vi "GoalieChute.vi"(6 "Current State":dbl=1.0, 8 "balls":T5[](array[typedef])=[{"x"=-974.5169677734375, "y"=-3444.3310546875, "timestamp"=timestamp(2082759045.994995 s since 1904-01-01), "Vel_x"=0.0, "Vel_y"=0.0}], 9 "Field Size in":T6={"line_width"=10, "field_length"=9000, "field_width"=6000, "boundary_width"=250, "referee_width"=425, "goal_width"=700, "goal_depth"=180, "goal_wall_width"=20, "center_circle_radius"=500, "defense_radius"=500, "defense_stretch"=350, "free_kick_from_defense_dist"=700, "penalty_spot_from_field_line_dist"=450, "penalty_line_from_spot_dist"=350}, 10 "Robot in":T2={"id"=5, "function"=enum."Attacker", "x"=-983.1382446289062, "y"=-3000.010498046875, "orientation"=-1.5516623258590698, "v_tangent"=0.0, "v_normal"=0.0, "v_ang"=0.0, "kick_x"=0.0, "kick_z"=0.0, "dribble"=FALSE, "Timestamp"=timestamp(2082759045.994995 s since 1904-01-01), "dest_x"=0.0, "dest_y"=0.0, "dest_orientation"=0.0, "estimatives"={"est_v_tangent"=0.0, "est_v_normal"=0.0, "est_vx"=0.0, "est_vy"=0.0}, "dest_x_kick"=0.0, "dest_y_kick"=0.0, "Gap Coord"=[], "States"=enum."GoToTangent"}, 11 "IA State Input 2":T1={"our_robots"=[], "enemy_robots"=[], "balls"=[], "geometry"={"line_width"=0, "field_length"=0, "field_width"=0, "boundary_width"=0, "referee_width"=0, "goal_width"=0, "goal_depth"=0, "goal_wall_width"=0, "center_circle_radius"=0, "defense_radius"=0, "defense_stretch"=0, "free_kick_from_defense_dist"=0, "penalty_spot_from_field_line_dist"=0, "penalty_line_from_spot_dist"=0}, "IA Judge"={"stage"="", "command"="", "our_goalie_id"=0.0, "enemy_goalie_id"=0.0, "command\nenum"=enum."Halt", "Time"=enum."Azul"}, "Received Timestamp"=timestamp(0 s since 1904-01-01), "Events"={"Touch"=FALSE, "Ball out"=FALSE, "id touch"=0.0, "Ball out of \nVision"=FALSE, "Ball inside \nGoalie area"=FALSE, "Robot not responding"=FALSE, "Robots responding status"=[1.0, 1.0, 1.0, 1.0, 1.0, 1.0], "Enemy Ball \nPossession"=FALSE}}) -> (1 "Next State":dbl=1.0, 2 "Robot out":T2={"id"=5, "function"=enum."Attacker", "x"=-983.1382446289062, "y"=-3000.010498046875, "orientation"=-1.5516623258590698, "v_tangent"=0.0001540345015520423, "v_normal"=0.008599927144915481, "v_ang"=0.002668461263266586, "kick_x"=0.0, "kick_z"=0.0, "dribble"=FALSE, "Timestamp"=timestamp(2082759045.994995 s since 1904-01-01), "dest_x"=0.0, "dest_y"=0.0, "dest_orientation"=0.0, "estimatives"={"est_v_tangent"=0.0, "est_v_normal"=0.0, "est_vx"=0.0, "est_vy"=0.0}, "dest_x_kick"=0.0, "dest_y_kick"=0.0, "Gap Coord"=[], "States"=enum."GoToTangent"})   [LabVIEW 2016]
uses:
  Core/AI Robot.ctl
  Functions Enum.ctl
  AttackerStates.ctl
  Core/Field Size.ctl
  Core/AI Ball.ctl
  Core/AI Input.ctl
  Core/AI Judge.ctl
  Command Enum.ctl
  <vilib>/Analysis/coordinate.llb/2D Cartesian Coordinate Rotation (Scalar).vi
  <vilib>/Analysis/NI_AALPro.lvlib
panel:
  out "V_tangent":dbl(graph)
  out "Waveform Chart":dbl(graph)
  out "Elapsed Time (s)":dbl
  in  "Time Target \nto transition":dbl=1.0 caption="Time Target (s)"
  in  "Longe":dbl=300.0 format="%#_13g"
  out "bola fora?":bool=TRUE
  in  "Cone de chute":dbl=0.09 format="%#_13g"
  in  "Perto":dbl=300.0 format="%#_13g"
  in  "Cone de rotação":dbl=1.3 format="%#_13g"
  in  "min dist to kick":dbl=150.0 format="%#_13g"
  in  "Dist a frente da bola":dbl format="%#_13g"
  in  "raio da circunferencia":dbl=175.0 format="%#_13g"
  in  "distance between ball and robot":dbl=125.0 format="%#_13g"
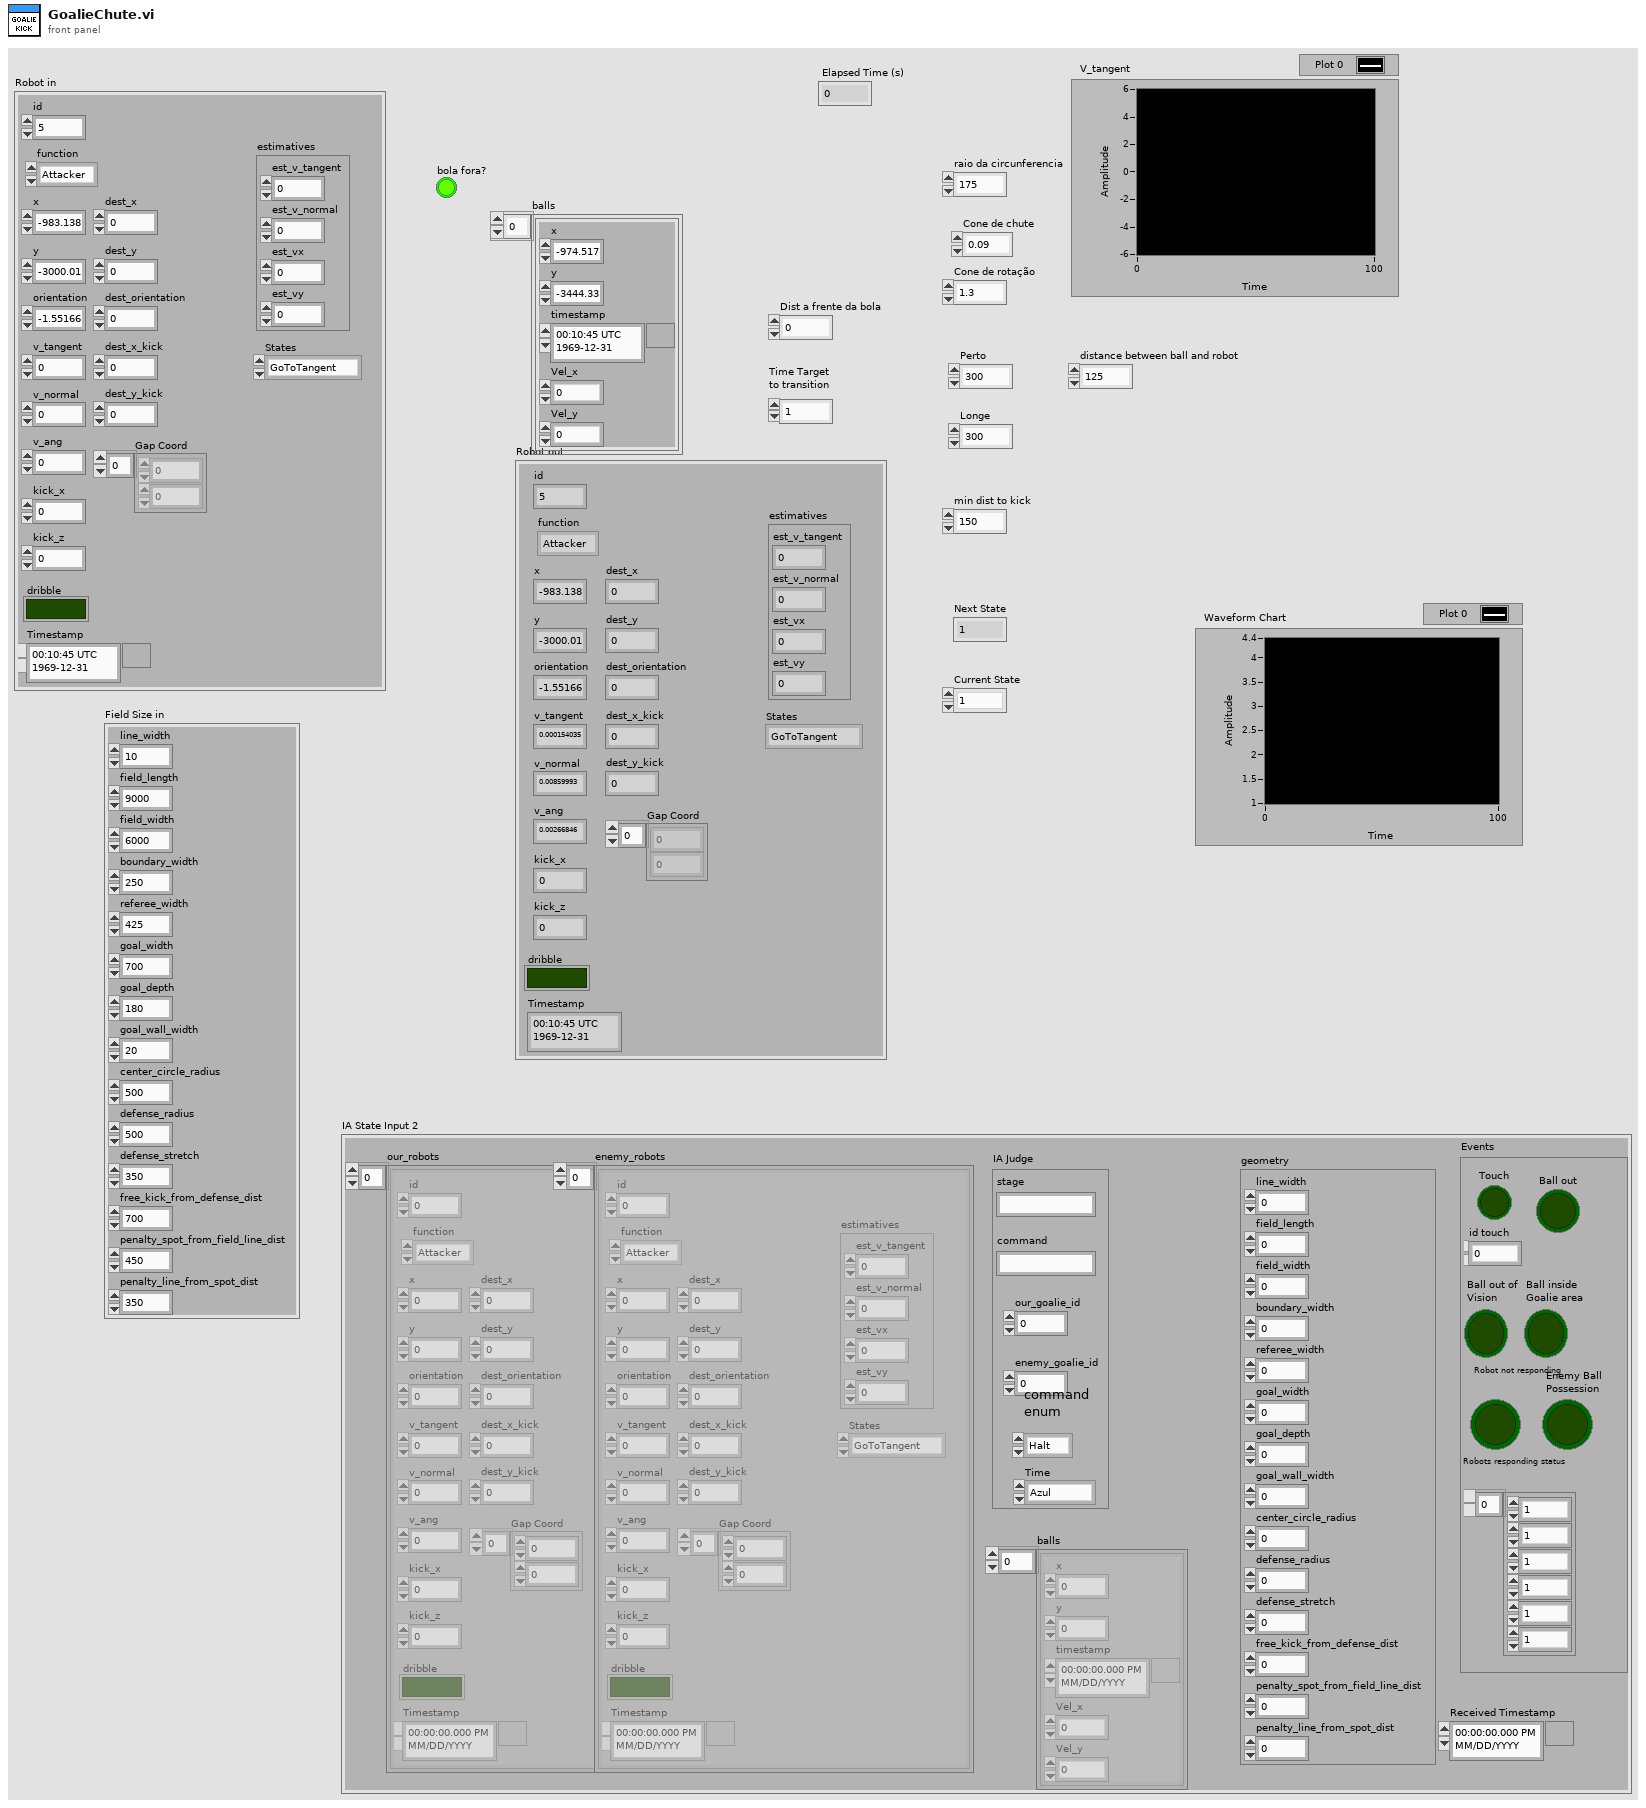
[diagram p1: front panel]
types:
  T1 = typedef "AI Input.ctl" = cluster{"our_robots":T2[], "enemy_robots":T2[], "balls":T5[], "geometry":T6, "IA Judge":T7, "Received Timestamp":timestamp, "Events":cluster{"Touch":bool, "Ball out":bool, "id touch":dbl, "Ball out of \nVision":bool, "Ball inside \nGoalie area":bool, "Robot not responding":bool, "Robots responding status":dbl[], "Enemy Ball \nPossession":bool}}
  T2 = typedef "AI Robot.ctl" = cluster{"id":u32, "function":T3, "x":dbl, "y":dbl, "orientation":dbl, "v_tangent":dbl, "v_normal":dbl, "v_ang":dbl, "kick_x":dbl, "kick_z":dbl, "dribble":bool, "Timestamp":timestamp, "dest_x":dbl, "dest_y":dbl, "dest_orientation":dbl, "estimatives":cluster{"est_v_tangent":dbl, "est_v_normal":dbl, "est_vx":dbl, "est_vy":dbl}, "dest_x_kick":dbl, "dest_y_kick":dbl, "Gap Coord":dbl[], "States":T4}
  T3 = typedef "Functions Enum.ctl" = enum16{"Attacker", "Goalie", "Defender", "Striker", "Goto 0", "Dummy", "Kicker", "ZigZag"}
  T4 = typedef "AttackerStates.ctl" = enum16{"Pass", "GoToTangent", "BallGetting", "GoToKick", ""}
  T5 = typedef "AI Ball.ctl" = cluster{"x":dbl, "y":dbl, "timestamp":timestamp, "Vel_x":dbl, "Vel_y":dbl}
  T6 = typedef "Field Size.ctl" = cluster{"line_width":u32, "field_length":u32, "field_width":u32, "boundary_width":u32, "referee_width":u32, "goal_width":u32, "goal_depth":u32, "goal_wall_width":u32, "center_circle_radius":u32, "defense_radius":u32, "defense_stretch":u32, "free_kick_from_defense_dist":u32, "penalty_spot_from_field_line_dist":u32, "penalty_line_from_spot_dist":u32}
  T7 = typedef "AI Judge.ctl" = cluster{"stage":string, "command":string, "our_goalie_id":dbl, "enemy_goalie_id":dbl, "command\nenum":T8, "Time":enum16{"Azul", "Amarelo"}}
  T8 = typedef "Command Enum.ctl" = enum16{"Halt", "Stop", "Force Start", "PKA Normal Start", "Prepare Kickoff Ally", "PKE Normal Start", "Prepare Kickoff Enemy", "Prepare Penalty Ally", "PPA Normal Start", "Prepare Penalty Enemy", "PPE Normal Start", "Direct Free Enemy", "Direct Free Ally", "Indirect Free Enemy", "Indirect Free Ally", "Timeout Enemy", "Timeout Ally", "Goal Enemy", "Goal Ally", "Ball Placement Enemy", "Ball Placement Ally", "Normal Half Time", "Extra Time Break", "Extra Half Time", "None"}
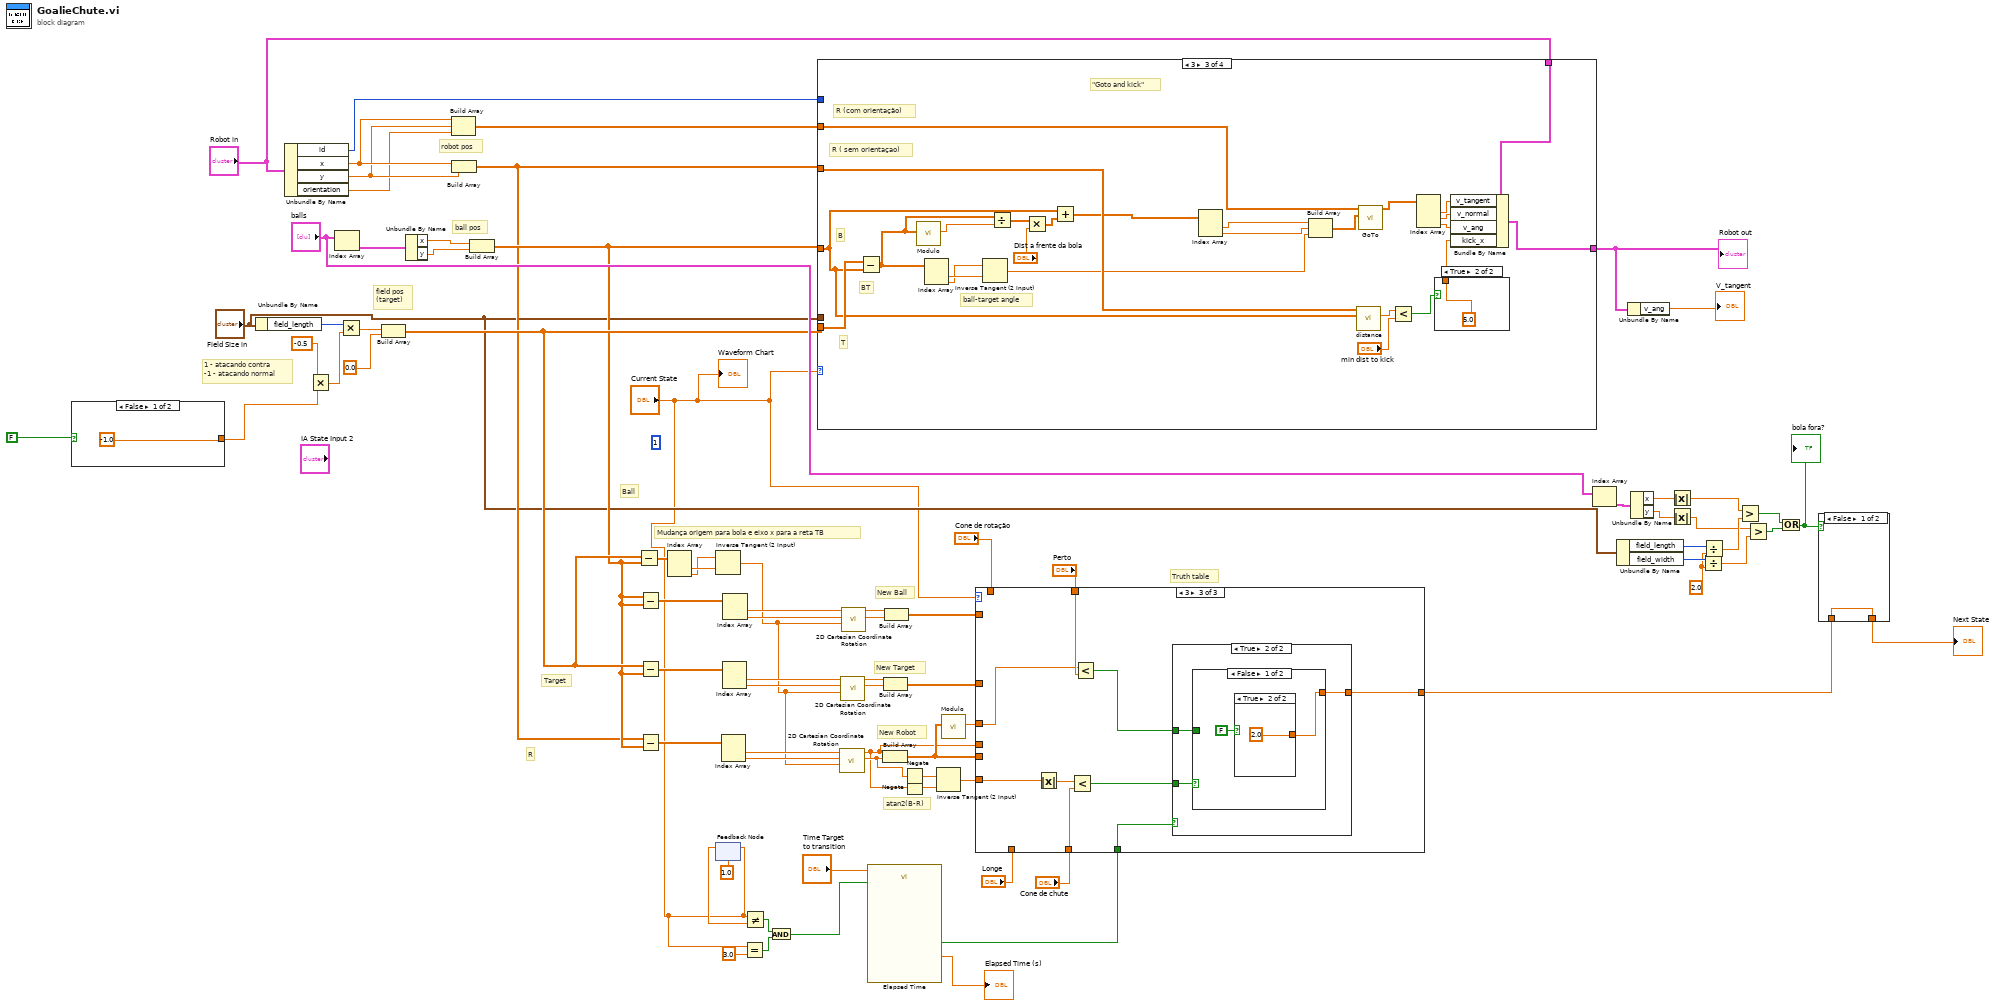
[diagram p0: block diagram]
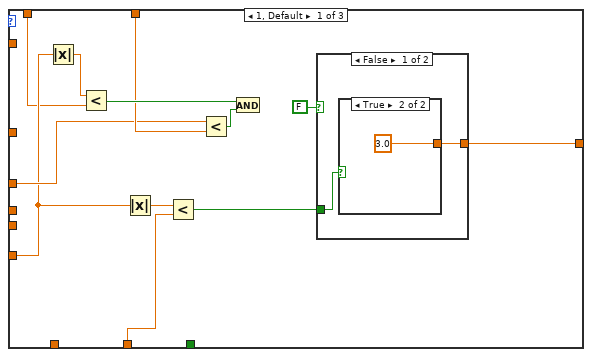
[diagram p2: hidden frame]
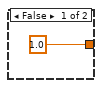
[diagram p3: hidden frame]
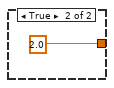
[diagram p4: hidden frame]
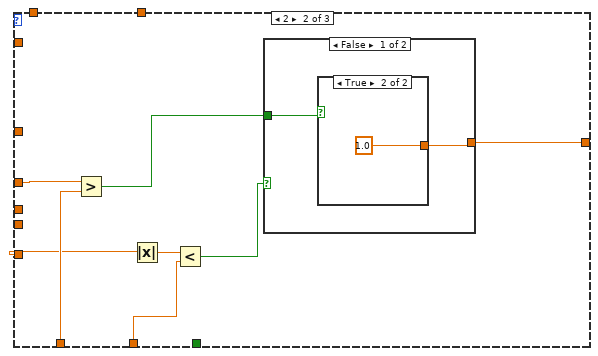
[diagram p5: hidden frame]
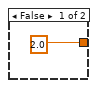
[diagram p6: hidden frame]
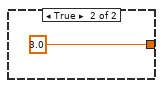
[diagram p7: hidden frame]
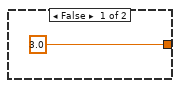
[diagram p8: hidden frame]
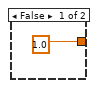
[diagram p9: hidden frame]
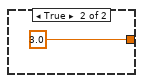
[diagram p10: hidden frame]
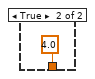
[diagram p11: hidden frame]
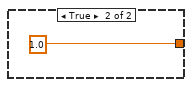
[diagram p12: hidden frame]
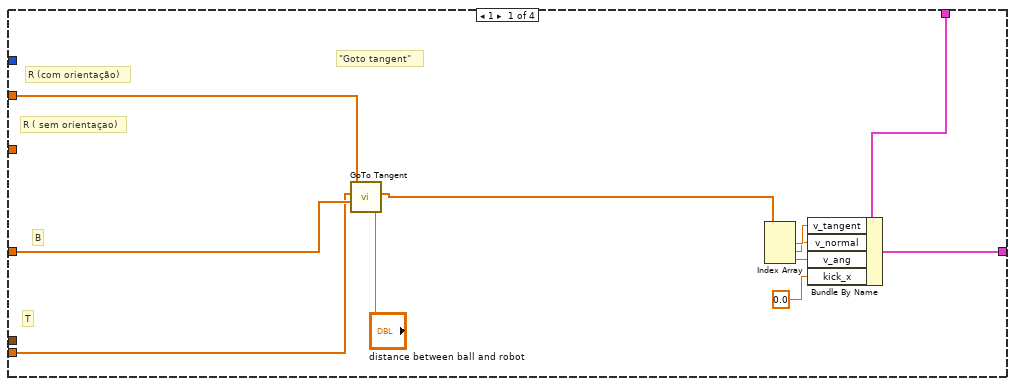
[diagram p13: hidden frame]
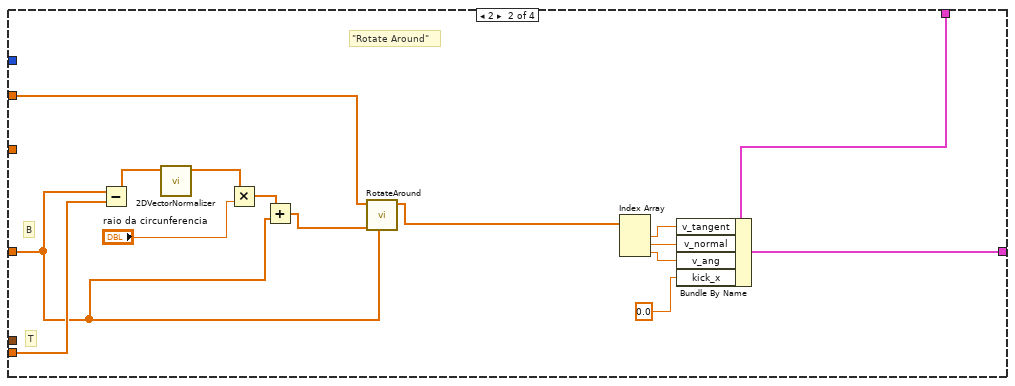
[diagram p14: hidden frame]
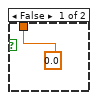
[diagram p15: hidden frame]
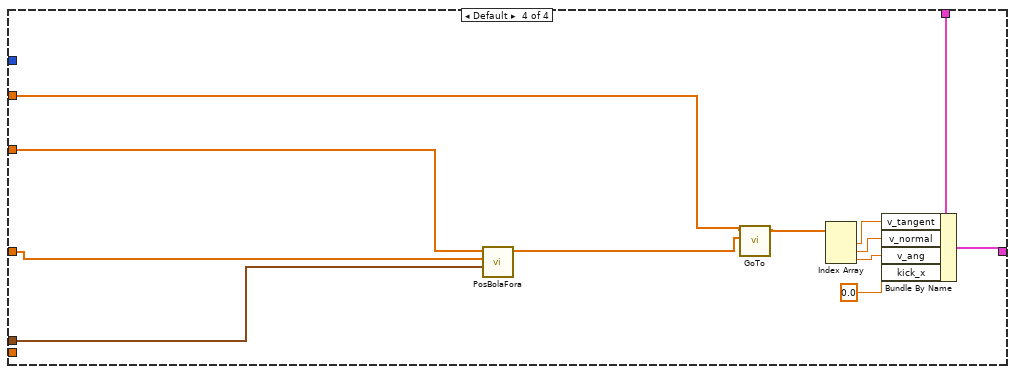
[diagram p16: hidden frame]
diagram:
  (unwired) 1
  w60 = 2.0 ("y")
  # "atan2(B-R)"
  # "New Robot"
  # "New Target"
  # "New Ball"
  # "R"
  # "Ball"
  # "Target"
  # "Mudança origem para bola e eixo x para a reta TB"
  # "1 - atacando contra\n-1 - atacando normal"
  # "Truth table"
  # "robot pos"
  # "field pos\n(target)"
  # "ball pos"
  n1 = case shown="False" FALSE {
    tunnel: [-1.0 ("attck contra? 2") 1.0] -> w22
    frame False {
    }
    frame True {
    }
  }
  n2 = Unbundle By Name("Field Size in") -> ("field_length"=w77:u32)
  n3 = Unbundle By Name("Robot in") -> ("id"=w16:u32, "x"=w73:dbl, "y"=w72:dbl, "orientation"=w69:dbl)
  n4 = Multiply(x=-0.5, y=w22) -> (x*y=w67:dbl)
  n5 = Index Array(array="balls") -> (element=w78:T5)  [unwired: 1 in]
  n6 = Multiply(x=w77, y=w67) -> (x*y=w76:dbl)
  n7 = Build Array(w76, 0.0 ("element")) -> (w34:dbl[])
  n8 = Unbundle By Name(w78) -> ("x"=w75:dbl, "y"=w74:dbl)
  n9 = Build Array(w73, w72, w69) -> (w70:dbl[])
  n10 = Build Array(w73, w72) -> (w32:dbl[])
  n11 = Build Array(w75, w74) -> (w33:dbl[])
  n12 = Subtract(x=w34, y=w33) -> (x-y=w42:dbl[])
  n13 = Subtract(x=w33, y=w33) -> (x-y=w49:dbl[])
  n14 = Subtract(x=w34, y=w33) -> (x-y=w46:dbl[])
  n15 = Subtract(x=w32, y=w33) -> (x-y=w43:dbl[])
  n16 = Index Array(array=w42) -> (element #1=w41:dbl, element #2=w40:dbl)  [unwired: 2 in]
  n17 = Inverse Tangent (2 Input)(1:w41, 2:w40) -> (0:w35:dbl)
  n18 = feedback #1(1.0 ("Current State")) -> (w8:dbl)
  n19 = feedback-in #1("Current State") -> ()
  n20 = Index Array(array=w43) -> (element #1=w45:dbl, element #2=w44:dbl)  [unwired: 2 in]
  n21 = Index Array(array=w46) -> (element #1=w48:dbl, element #2=w47:dbl)  [unwired: 2 in]
  n22 = Index Array(array=w49) -> (element #1=w51:dbl, element #2=w50:dbl)  [unwired: 2 in]
  n23 = Equal?(x="Current State", y=3.0) -> (x = y?=w12:bool)
  n24 = Not Equal?(x="Current State", y=w8) -> (x != y?=w11:bool)
  n25 = And(x=w11, y=w12) -> (x .and. y?=w6:bool)
  n26 = case shown="3" "Current State" {
    tunnel: [w91 w106 w132 w146] -> w4
    tunnel: "Robot in" -> [w90 w93 w131 w145]
    tunnel: w70 -> [w88 w105 w117 w137]
    tunnel: w32 -> [_ _ w126 w139]
    tunnel: w33 -> [w84 w92 w107 w140]
    tunnel: w34 -> [w83 w99 w123 _]
    tunnel: "Field Size in" -> [_ _ _ w138]
    tunnel: w16 -> [_ _ _ _]
    frame 1 {
      # "\"Goto tangent\""
      # "B"
      # "T"
      # "R ( sem orientaçao)"
      # "R (com orientação)"
      n27 = call "GoTo Tangent.vi"("distance between ball and robot"="distance between ball and robot", "Ball"=w84, "Target"=w83, "R"=w88) -> ("Output\nVelocity"=w82:dbl[])  [unwired: 6 in, 1 out]
      n28 = Index Array(array=w82) -> (element #1=w87:dbl, element #2=w86:dbl, element #3=w85:dbl)  [unwired: 3 in]
      n29 = Bundle By Name(cluster=w90, "v_tangent"=w87, "v_normal"=w86, "v_ang"=w85, "kick_x"=0.0) -> (w91:T2)
    }
    frame 2 {
      # "T"
      # "B"
      # "\"Rotate Around\""
      n30 = Subtract(x=w92, y=w99) -> (x-y=w98:dbl[])
      n31 = call "2DVectorNormalizer.vi"("2D vector"=w98) -> ("2D vector 2"=w97:dbl[])  [unwired: 10 in]
      n32 = Multiply(x=w97, y="raio da circunferencia") -> (x*y=w95:dbl[])
      n33 = Add(x=w95, y=w92) -> (x+y=w94:dbl[])
      n34 = call "RotateAround.vi"("Centre"=w92, "Target"=w94, "Position"=w105) -> ("Output\nVelocity"=w100:dbl[])  [unwired: 8 in]
      n35 = Index Array(array=w100) -> (element #1=w103:dbl, element #2=w102:dbl, element #3=w101:dbl)  [unwired: 3 in]
      n36 = Bundle By Name(cluster=w93, "v_tangent"=w103, "v_normal"=w102, "v_ang"=w101, "kick_x"=0.0) -> (w106:T2)
    }
    frame 3 {
      # "BT"
      # "ball-target angle"
      # "B"
      # "T"
      # "R ( sem orientaçao)"
      # "R (com orientação)"
      # "\"Goto and kick\""
      n37 = Subtract(x=w123, y=w107) -> (x-y=w108:dbl[])
      n38 = call "Modulo.vi"("2D vector"=w108) -> ("Modulo"=w109:dbl)  [unwired: 10 in]
      n39 = Index Array(array=w108) -> (element #1=w125:dbl, element #2=w124:dbl)  [unwired: 2 in]
      n40 = Inverse Tangent (2 Input)(1:w125, 2:w124) -> (0:w122:dbl)
      n41 = Divide(x=w108, y=w109) -> (x/y=w110:dbl[])
      n42 = Multiply(x=w110, y="Dist a frente da bola") -> (x*y=w113:dbl[])
      n43 = Add(x=w107, y=w113) -> (x+y=w111:dbl[])
      n44 = Index Array(array=w111) -> (element #1=w121:dbl, element #2=w120:dbl)  [unwired: 2 in]
      n45 = Build Array(w121, w120, w122) -> (w119:dbl[])
      n46 = call "distance.vi"("target pos"=w107, "obj pos"=w126) -> ("sqrt(x)"=w130:dbl)  [unwired: 9 in]
      n47 = call "GoTo.vi"("Target"=w119, "Position"=w117) -> ("Output\nVelocity"=w118:dbl[])  [unwired: 8 in, 1 out]
      n48 = Less?(x=w130, y="min dist to kick") -> (x < y?=w128:bool)
      n49 = Index Array(array=w118) -> (element #1=w116:dbl, element #2=w115:dbl, element #3=w114:dbl)  [unwired: 3 in]
      n50 = case shown="True" w128 {
        tunnel: [0.0 5.0] -> w129
        frame False {
        }
        frame True {
        }
      }
      n51 = Bundle By Name(cluster=w131, "v_tangent"=w116, "v_normal"=w115, "v_ang"=w114, "kick_x"=w129) -> (w132:T2)
    }
    frame Default {
      n52 = call "PosBolaFora.vi"("Field Size in"=w138, "Position da bola"=w140, "Position do robot"=w139) -> ("Target"=w136:dbl[])  [unwired: 8 in]
      n53 = call "GoTo.vi"("Target"=w136, "Position"=w137) -> ("Output\nVelocity"=w135:dbl[])  [unwired: 8 in, 1 out]
      n54 = Index Array(array=w135) -> (element #1=w143:dbl, element #2=w142:dbl, element #3=w141:dbl)  [unwired: 3 in]
      n55 = Bundle By Name(cluster=w145, "v_tangent"=w143, "v_normal"=w142, "v_ang"=w141, "kick_x"=0.0) -> (w146:T2)
    }
  }
  "Robot out" <- w4
  n56 = call-poly <vilib>:"2D Cartesian Coordinate Rotation.vi"("theta"=w35, "y"=w44, "x"=w45) -> ("y out"=w19:dbl, "x out"=w18:dbl)  [unwired: 6 in, 1 out]
  n57 = call-poly <vilib>:"2D Cartesian Coordinate Rotation.vi"("theta"=w35, "y"=w47, "x"=w48) -> ("y out"=w38:dbl, "x out"=w39:dbl)  [unwired: 6 in, 1 out]
  n58 = call-poly <vilib>:"2D Cartesian Coordinate Rotation.vi"("theta"=w35, "y"=w50, "x"=w51) -> ("y out"=w36:dbl, "x out"=w37:dbl)  [unwired: 6 in, 1 out]
  n59 = call "Elapsed Time"("Time Target (s)"="Time Target \nto transition", "Reset"=w6) -> ("Elapsed Time (s)"=→"Elapsed Time (s)":dbl, "Time has Elapsed"=w14:bool)  [unwired: 10 in, 6 out]
  n60 = Build Array(w18, w19) -> (w27:dbl[])
  n61 = Build Array(w39, w38) -> (w28:dbl[])
  n62 = Build Array(w37, w36) -> (w29:dbl[])
  n63 = Negate(x=w19) -> (-x=w21:dbl)
  n64 = Negate(x=w18) -> (-x=w20:dbl)
  n65 = Inverse Tangent (2 Input)(1:w20, 2:w21) -> (0:w25:dbl)
  n66 = call "Modulo.vi"("2D vector"=w27) -> ("Modulo"=w26:dbl)  [unwired: 10 in]
  n67 = case shown="3" "Current State" {
    tunnel: "Longe" -> [_ w170 _]
    tunnel: "Cone de chute" -> [w152 w165 w180]
    tunnel: w29 -> [_ _ _]
    tunnel: w28 -> [_ _ _]
    tunnel: w27 -> [_ _ _]
    tunnel: w26 -> [w155 w171 w183]
    tunnel: w25 -> [w150 w166 w181]
    tunnel: [w154 w169 w185] -> w24
    tunnel: "Perto" -> [w156 _ w184]
    tunnel: w18 -> [_ _ _]
    tunnel: w14 -> [_ _ w177]
    tunnel: "Cone de rotação" -> [w148 _ _]
    frame 1, Default {
      n68 = Absolute Value(x=w150) -> (abs(x)=w149:dbl)
      n69 = Less?(x=w149, y=w148) -> (x < y?=w158:bool)
      n70 = Absolute Value(x=w150) -> (abs(x)=w153:dbl)
      n71 = Less?(x=w153, y=w152) -> (x < y?=w151:bool)
      n72 = Less?(x=w155, y=w156) -> (x < y?=w157:bool)
      n73 = And(x=w158, y=w157) -> ()  [unwired: 1 out]
      n74 = case shown="False" FALSE {
        tunnel: [w160 2.0] -> w154
        tunnel: w151 -> [w159 _]
        frame False {
          n75 = case shown="True" w159 {
            tunnel: [1.0 3.0] -> w160
            frame False {
            }
            frame True {
            }
          }
        }
        frame True {
        }
      }
    }
    frame 2 {
      n76 = Greater?(x=w171, y=w170) -> (0:w168:bool)
      n77 = Absolute Value(x=w166) -> (abs(x)=w167:dbl)
      n78 = Less?(x=w167, y=w165) -> (x < y?=w164:bool)
      n79 = case shown="False" w164 {
        tunnel: [w172 3.0] -> w169
        tunnel: w168 -> [w173 _]
        frame False {
          n80 = case shown="True" w173 {
            tunnel: [2.0 1.0] -> w172
            frame False {
            }
            frame True {
            }
          }
        }
        frame True {
        }
      }
    }
    frame 3 {
      n81 = Absolute Value(x=w181) -> (abs(x)=w182:dbl)
      n82 = Less?(x=w182, y=w180) -> (x < y?=w179:bool)
      n83 = Less?(x=w183, y=w184) -> (x < y?=w178:bool)
      n84 = case shown="True" w177 {
        tunnel: [3.0 w189] -> w185
        tunnel: w179 -> [_ w188]
        tunnel: w178 -> [_ w187]
        frame False {
        }
        frame True {
          n85 = case shown="False" w188 {
            tunnel: [w191 3.0] -> w189
            tunnel: w187 -> [_ _]
            frame False {
              n86 = case shown="True" FALSE {
                tunnel: [1.0 2.0] -> w191
                frame False {
                }
                frame True {
                }
              }
            }
            frame True {
            }
          }
        }
      }
    }
  }
  n87 = Index Array(array="balls") -> (element=w65:T5)  [unwired: 1 in]
  n88 = Unbundle By Name("Field Size in") -> ("field_length"=w62:u32, "field_width"=w61:u32)
  n89 = Unbundle By Name(w4) -> ("v_ang"=→"V_tangent":dbl)
  n90 = Unbundle By Name(w65) -> ("x"=w64:dbl, "y"=w63:dbl)
  n91 = Absolute Value(x=w64) -> (abs(x)=w59:dbl)
  n92 = Absolute Value(x=w63) -> (abs(x)=w57:dbl)
  n93 = Divide(x=w61, y=w60) -> (x/y=w56:dbl)
  n94 = Divide(x=w62, y=w60) -> (x/y=w58:dbl)
  n95 = Greater?(x=w59, y=w58) -> (0:w55:bool)
  n96 = Greater?(x=w57, y=w56) -> (0:w54:bool)
  n97 = Or(x=w55, y=w54) -> (x .or. y?=w53:bool)
  "bola fora?" <- w53
  n98 = case shown="False" w53 {
    tunnel: [w195 4.0] -> w9
    tunnel: w24 -> [w195 _]
    frame False {
    }
    frame True {
    }
  }
  "Next State" <- w9
  "Waveform Chart" <- "Current State"
